vi "Cal Interpolation_2.vi"() -> ()   [LabVIEW 2018]
doc: "This example shows the operation of the 1D interpolation VI using three selectable test sets."
uses:
  <vilib>/gmath/NI_Gmath.lvlib
  <vilib>/Utility/file.llb/Read From Spreadsheet File (DBL).vi
panel:
  in  "all rows":dbl[][](array[numeric])=[[50000000.0, 100000000.0, 150000000.0, 200000000.0, 250000000.0, 300000000.0, 350000000.0, 400000000.0, 450000000.0, 500000000.0, 550000000.0, 600000000.0, 650000000.0, 700000000.0, 750000000.0, 800000000.0, 850000000.0, 900000000.0, 950000000.0, 1000000000.0, 1050000000.0, 1100000000.0, 1150000000.0, 1200000000.0, 1250000000.0, 1300000000.0, 1350000000.0, 1400000000.0, 1450000000.0, 1500000000.0, 1550000000.0, 1600000000.0, 1650000000.0, 1700000000.0, 1750000000.0, 1800000000.0, 1850000000.0, 1900000000.0, 1950000000.0, 2000000000.0, 2050000000.0, 2100000000.0, 2150000000.0, 2200000000.0, 2250000000.0, 2300000000.0, 2350000000.0, 2400000000.0, 2450000000.0, 2500000000.0, 2550000000.0, 2600000000.0, 2650000000.0, 2700000000.0, 2750000000.0, 2800000000.0, 2850000000.0, 2900000000.0, 2950000000.0, 3000000000.0], [-0.08, -0.16, -0.21, -0.23, -0.24, -0.28, -0.3, -0.34, -0.33, -0.31, -0.38, -0.37, -0.42, -0.39, -0.48, -0.41, -0.45, -0.41, -0.46, -0.48, -0.53, -0.57, -0.58, -0.65, -0.6, -0.71, -0.66, -0.77, -0.68, -0.78, -0.76, -0.88, -0.81, -0.83, -0.87, -0.83, -0.97, -0.81, -0.92, -0.79, -1.11, -0.76, -0.94, -0.98, -1.08, -0.9, -0.89, -1.14, -1.07, -1.25, -0.93, -1.25, -0.97, -1.38, -1.03, -1.17, -1.06, -1.21, -1.13, -0.98], [-6.65, -6.76, -6.93, -7.18, -7.18, -7.1, -7.38, -7.15, -7.28, -7.26, -7.24, -7.2, -7.36, -7.25, -7.49, -7.47, -7.53, -7.51, -7.88, -7.68, -7.97, -7.71, -7.89, -7.81, -7.91, -7.86, -7.94, -7.9, -7.97, -8.04, -8.08, -8.0, -8.12, -8.12, -8.29, -8.21, -8.41, -8.33, -8.43, -8.28, -8.91, -8.32, -8.78, -8.53, -8.99, -8.69, -8.98, -8.66, -9.24, -8.98, -8.95, -9.08, -9.02, -9.57, -9.73, -10.52, -10.26, -12.76, -13.4, -16.45], [-6.86, -6.86, -6.91, -7.31, -7.13, -7.12, -7.41, -7.13, -7.26, -7.16, -7.21, -7.16, -7.28, -7.19, -7.36, -7.35, -7.47, -7.41, -7.71, -7.57, -7.84, -7.64, -7.81, -7.77, -7.76, -7.89, -7.87, -7.94, -7.84, -8.05, -8.02, -8.06, -8.05, -8.14, -8.3, -8.19, -8.41, -8.36, -8.48, -8.27, -8.95, -8.31, -8.81, -8.49, -8.91, -8.64, -8.83, -8.49, -9.03, -8.8, -8.69, -8.97, -8.8, -9.38, -9.57, -10.78, -10.64, -12.82, -14.4, -17.28], [-0.19, -0.304, -0.304, -0.351, -0.339, -0.296, -0.371, -0.336, -0.432, -0.473, -0.503, -0.432, -0.446, -0.458, -0.627, -0.623, -0.587, -0.637, -0.778, -0.751, -0.707, -0.637, -0.654, -0.623, -0.707, -0.721, -0.778, -0.694, -0.707, -0.821, -0.991, -0.963, -0.778, -0.666, -0.749, -0.963, -1.093, -0.934, -0.877, -0.877, -1.05, -1.056, -0.892, -0.764, -0.877, -1.124, -1.272, -1.166, -1.05, -1.006, -1.008, -1.256, -1.345, -1.05, -1.008, -1.333, -1.516, -1.087, -1.124, -1.331]]
  in  "Freq Select":dbl=51000000.0
  out "Last Ofs Value":dbl
  out "Next Ofs Value":dbl
  out "Orig Ofs Data":dbl[](array[numeric])
  out "Next Freq Value":dbl
  out "Last Freq Value":dbl
  out "Orig Freq data":dbl[](array[numeric])
  out "size(s)":i32[](array[numeric])=[295001, 2]
  in  "INst":i32=1
  in  "Tab Control":enum32{"Graph", "Data"}(tab)
  out "1D Interpolation Graph":cluster{"yi":dbl[], "ramp data":dbl[]}[](graph)=[{"yi"=[50000000.0, 100000000.0, 150000000.0, 200000000.0, 250000000.0, 300000000.0, 350000000.0, 400000000.0, 450000000.0, 500000000.0, 550000000.0, 600000000.0, 650000000.0, 700000000.0, 750000000.0, 800000000.0, 850000000.0, 900000000.0, 950000000.0, 1000000000.0, 1050000000.0, 1100000000.0, 1150000000.0, 1200000000.0, 1250000000.0, 1300000000.0, 1350000000.0, 1400000000.0, 1450000000.0, 1500000000.0, 1550000000.0, 1600000000.0, 1650000000.0, 1700000000.0, 1750000000.0, 1800000000.0, 1850000000.0, 1900000000.0, 1950000000.0, 2000000000.0, 2050000000.0, 2100000000.0, 2150000000.0, 2200000000.0, 2250000000.0, 2300000000.0, 2350000000.0, 2400000000.0, 2450000000.0, 2500000000.0, 2550000000.0, 2600000000.0, 2650000000.0, 2700000000.0, 2750000000.0, 2800000000.0, 2850000000.0, 2900000000.0, 2950000000.0, 3000000000.0], "ramp data"=[-0.08, -0.16, -0.21, -0.23, -0.24, -0.28, -0.3, -0.34, -0.33, -0.31, -0.38, -0.37, -0.42, -0.39, -0.48, -0.41, -0.45, -0.41, -0.46, -0.48, -0.53, -0.57, -0.58, -0.65, -0.6, -0.71, -0.66, -0.77, -0.68, -0.78, -0.76, -0.88, -0.81, -0.83, -0.87, -0.83, -0.97, -0.81, -0.92, -0.79, -1.11, -0.76, -0.94, -0.98, -1.08, -0.9, -0.89, -1.14, -1.07, -1.25, -0.93, -1.25, -0.97, -1.38, -1.03, -1.17, -1.06, -1.21, -1.13, -0.98]}, {"yi"=array[295001 elements], "ramp data"=array[295001 elements]}]
  out "Interpolated Data":dbl[][](array[numeric])
  out "Original Data":dbl[][](array[numeric])=[[50000000.0, -0.08], [100000000.0, -0.16], [150000000.0, -0.21], [200000000.0, -0.23], [250000000.0, -0.24], [300000000.0, -0.28], [350000000.0, -0.3], [400000000.0, -0.34], [450000000.0, -0.33], [500000000.0, -0.31], [550000000.0, -0.38], [600000000.0, -0.37], [650000000.0, -0.42], [700000000.0, -0.39], [750000000.0, -0.48], [800000000.0, -0.41], [850000000.0, -0.45], [900000000.0, -0.41], [950000000.0, -0.46], [1000000000.0, -0.48], [1050000000.0, -0.53], [1100000000.0, -0.57], [1150000000.0, -0.58], [1200000000.0, -0.65], [1250000000.0, -0.6], [1300000000.0, -0.71], [1350000000.0, -0.66], [1400000000.0, -0.77], [1450000000.0, -0.68], [1500000000.0, -0.78], [1550000000.0, -0.76], [1600000000.0, -0.88], [1650000000.0, -0.81], [1700000000.0, -0.83], [1750000000.0, -0.87], [1800000000.0, -0.83], [1850000000.0, -0.97], [1900000000.0, -0.81], [1950000000.0, -0.92], [2000000000.0, -0.79], [2050000000.0, -1.11], [2100000000.0, -0.76], [2150000000.0, -0.94], [2200000000.0, -0.98], [2250000000.0, -1.08], [2300000000.0, -0.9], [2350000000.0, -0.89], [2400000000.0, -1.14], [2450000000.0, -1.07], [2500000000.0, -1.25], [2550000000.0, -0.93], [2600000000.0, -1.25], [2650000000.0, -0.97], [2700000000.0, -1.38], [2750000000.0, -1.03], [2800000000.0, -1.17], [2850000000.0, -1.06], [2900000000.0, -1.21], [2950000000.0, -1.13], [3000000000.0, -0.98]]
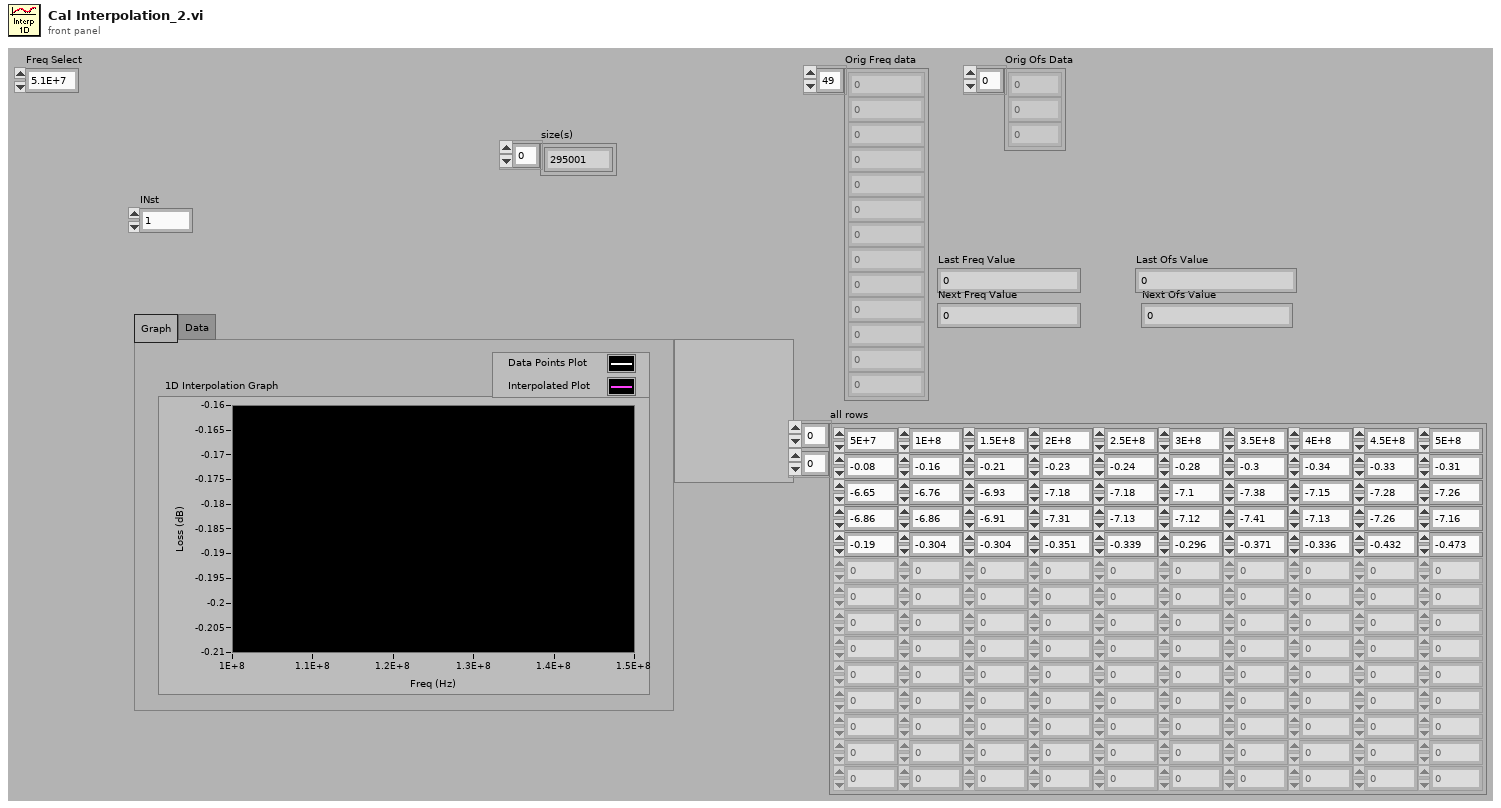
[diagram p1: front panel]
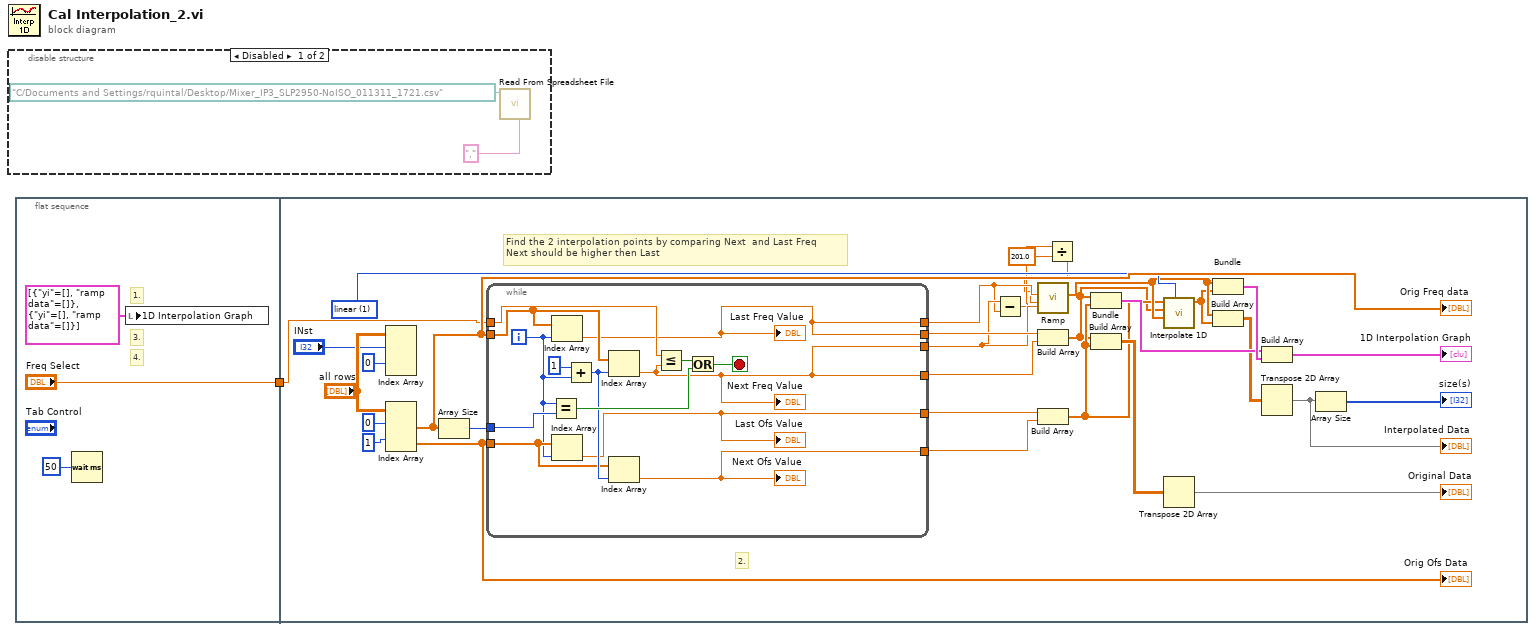
[diagram p0: block diagram]
diagram:
  n1 = disable-structure shown="Disabled" {
    frame Disabled {
      n2 = call-poly <vilib>:"Read From Spreadsheet File.vi"("delimiter (\\t)"="," ("delimiter (\\t)"), "file path (dialog if empty)"=path "C:/Documents and Settings/rquintal/Desktop/Mixer_IP3_SLP2950-NoISO_011311_1721.csv") -> ()  [unwired: 5 in, 5 out]
    }
    frame Enabled {
    }
  }
  n3 = flat-sequence {
    tunnel: ["Freq Select"] -> w1
    tunnel: w1 -> [w12]
    frame #0 {
      # "4."
      # "3."
      # "1."
      n4 = Wait (ms)(milliseconds to wait=u32 50) -> ()  [unwired: 1 out]
      n5 = local write "1D Interpolation Graph"(cluster{"yi":i32[], "ramp data":i32[]}[] [{"yi"=[], "ramp data"=[]}, {"yi"=[], "ramp data"=[]}] ("1D Interpolation Graph")) -> ()
    }
    frame #1 {
      w31 = 1 items=["nearest", "linear", "spline", "cubic Hermite", "Lagrange"] ("Method")
      # "Find the 2 interpolation points by comparing Next  and Last Freq\nNext should be higher then Last"
      # "2."
      n6 = Index Array(array="all rows", index (row) #1="INst", index (row) #2=0 ("index (row)")) -> ()  [unwired: 2 in, 2 out]
      n7 = Index Array(array="all rows", index (row) #1=0 ("index (row)"), index (row) #2=1 ("index (row)")) -> (element #1=w35:dbl[], element #2=w17:dbl[])  [unwired: 2 in]
      "Orig Freq data" <- w35
      "Orig Ofs Data" <- w17
      n8 = Array Size(array=w35) -> (size(s)=w34:i32)
      n9 = while {
        tunnel: w35 -> [w50]
        tunnel: w34 -> [w49]
        tunnel: w12 -> [w48]
        tunnel: [w39] -> w33
        tunnel: [w38] -> w32
        tunnel: w17 -> [w43]
        tunnel: [w41] -> w16
        tunnel: [w40] -> w15
        tunnel: [w39] -> w10
        tunnel: [w38] -> w11
        i -> [w42]
        stop <- w46 stop-if-true
        n10 = Equal?(x=w42, y=w49) -> (x = y?=w47:bool)
        n11 = Index Array(array=w50, index=w42) -> (element=w39:dbl)
        "Last Freq Value" <- w39
        n12 = Index Array(array=w43, index=w42) -> (element=w41:dbl)
        "Last Ofs Value" <- w41
        n13 = Add(x=1, y=w42) -> (x+y=w44:i32)
        n14 = Index Array(array=w50, index=w44) -> (element=w38:dbl)
        "Next Freq Value" <- w38
        n15 = Index Array(array=w43, index=w44) -> (element=w40:dbl)
        "Next Ofs Value" <- w40
        n16 = Less Or Equal?(x=w48, y=w38) -> (x <= y?=w45:bool)
        n17 = Or(x=w45, y=w47) -> (x .or. y?=w46:bool)
      }
      n18 = Subtract(x=w11, y=w10) -> (x-y=w9:dbl)
      n19 = Build Array(w33, w32) -> (w13:dbl[])
      n20 = Build Array(w16, w15) -> (w14:dbl[])
      n21 = Divide(x=w9, y=201.0) -> (x/y=w7:dbl)
      n22 = call "Ramp.vi"("# of Samples"=w11, "Start"=w7, "Stop"=w10) -> ("Output"=w24:dbl[])  [unwired: 8 in]
      n23 = Bundle(w13, w14) -> (w28:cluster{dbl[], dbl[]})  [unwired: 1 in]
      n24 = Build Array(w13, w14) -> (w27:dbl[][])
      n25 = call <vilib>:"Interpolate 1D.vi"("method"=w31, "xi"=w24, "X"=w13, "Y"=w14) -> ("yi"=w23:dbl[])  [unwired: 5 in, 2 out]
      n26 = Transpose 2D Array(2D array=w27) -> (transposed array=→"Original Data":dbl[][])
      n27 = Bundle("Output"=w24, "yi"=w23) -> (w29:cluster{"Output":dbl[], "yi":dbl[]})  [unwired: 1 in]
      n28 = Build Array(w24, w23) -> (w25:dbl[][])
      n29 = Build Array(w28, w29) -> (→"1D Interpolation Graph":cluster{"Output":dbl[], "yi":dbl[]}[])
      n30 = Transpose 2D Array(2D array=w25) -> (transposed array=w20:dbl[][])
      "Interpolated Data" <- w20
      n31 = Array Size(array=w20) -> (size(s)=→"size(s)":i32[])
    }
  }
